vi "Set API.vi"(8 "error in (no error)":errorcluster, 10 "Actor API":refnum<class "Actor API.lvclass">, 11 "Actor in":refnum<class "Actor.lvclass">) -> (0 "error out":errorcluster, 3 "Actor out":refnum<class "Actor.lvclass">)   [LabVIEW 2020, in "Artifex.lvlib" / "Actor.lvclass"]
uses:
  Actor.lvclass
  Actor Proxy/Actor API.lvclass
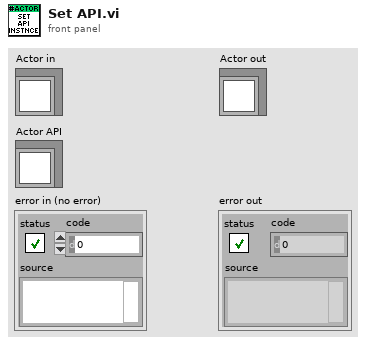
[diagram p1: front panel]
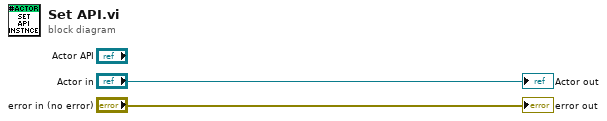
[diagram p0: block diagram]
diagram:
  "error out" <- "error in (no error)"
  "Actor out" <- "Actor in"
